vi "Main.vi"() -> ()   [LabVIEW 2017]
uses:
  classes/Scans/Scan.lvclass
  classes/HardwareObjects/DAQ/DAQ.lvclass/DAQ.ctl
  classes/HardwareObjects/Galvonometer/Galvonometer.lvclass/Galvonometer.ctl
  classes/HardwareObjects/Camera/Camera.lvclass/Camera.ctl
  classes/HardwareObjects/PC/PC.lvclass/PC.ctl
  classes/HardwareObjects/Spectrometer/Spectrometer.lvclass/Spectrometer.ctl
  classes/SoftwareObjects/ConfigProc/ConfigProc.lvclass/ConfigProc.ctl
  classes/Scans/Scan.lvclass/Scan.ctl
  classes/HardwareObjects/DAQ/Write Galvo Analog Output Channel(s).vi
  classes/HardwareObjects/Galvonometer/Write Analog Output Channel.vi
  classes/HardwareObjects/Galvonometer/Write Scan Direction.vi
  classes/HardwareObjects/Camera/Write Bit Depth.vi
  classes/HardwareObjects/Camera/Write Camera Dimensions.vi
  classes/HardwareObjects/Camera/Write Data Representation.vi
  classes/HardwareObjects/Camera/Write Duty Cycle.vi
  classes/HardwareObjects/Camera/Write Make, Model.vi
  classes/HardwareObjects/Camera/Write Max Frequency (kHz).vi
  classes/HardwareObjects/Camera/Write Return Time (us).vi
  classes/HardwareObjects/PC/Write Max Number of Cores.vi
  classes/HardwareObjects/PC/Write Path to DLL.vi
  classes/HardwareObjects/DAQ/Write Camera Counter.vi
  classes/HardwareObjects/DAQ/Write Camera Counter Output Terminal.vi
  classes/HardwareObjects/DAQ/Write Galvo Counter.vi
  classes/HardwareObjects/DAQ/Write Galvo Counter Terminal.vi
  classes/HardwareObjects/DAQ/Write Master Counter.vi
  classes/HardwareObjects/DAQ/Write Master Counter Terminal.vi
  classes/HardwareObjects/Spectrometer/Write Bandwidth (nm).vi
  classes/HardwareObjects/Spectrometer/Write Center wavelength (nm).vi
  classes/HardwareObjects/Spectrometer/Write Make Model.vi
  classes/HardwareObjects/Spectrometer/Write Scan depth (mm).vi
  classes/HardwareObjects/Galvonometer/Write Make Model.vi
  classes/HardwareObjects/Galvonometer/Write Max Scan Angle (degrees).vi
  classes/HardwareObjects/Galvonometer/Write Output Scale Factor (V_degrees).vi
  classes/SoftwareObjects/ConfigProc/Write Blur Coefficient.vi
  classes/SoftwareObjects/ConfigProc/Write Blur Int.vi
  classes/SoftwareObjects/ConfigProc/Write Cores.vi
  classes/SoftwareObjects/ConfigProc/Write Interpolation.vi
  classes/SoftwareObjects/ConfigProc/Write Magnification.vi
  classes/SoftwareObjects/ConfigProc/Write Power.vi
  classes/SoftwareObjects/ConfigProc/Write Soften.vi
  classes/Scans/Read X FOV (degrees).vi
  classes/Scans/Read Y FOV (degrees).vi
  classes/HardwareObjects/DAQ/DAQ.lvclass
  classes/HardwareObjects/Galvonometer/Galvonometer.lvclass
  classes/HardwareObjects/Camera/Camera.lvclass
  classes/HardwareObjects/PC/PC.lvclass
  classes/HardwareObjects/Spectrometer/Spectrometer.lvclass
  classes/SoftwareObjects/ConfigProc/ConfigProc.lvclass
panel:
  out "P":dbl[](array[numeric])=[1.0, 2.0, 3.0, 4.0, 5.0, 6.0, 7.0, 8.0, 9.0, 10.0, 11.0, 12.0, 13.0, 14.0, 15.0, 16.0, 17.0, 18.0, 19.0, 20.0, 21.0, 22.0, 23.0, 24.0, 25.0, 26.0, 27.0, 28.0, 29.0, 30.0, 31.0, 32.0, 33.0, 34.0, 35.0, 36.0, 37.0, 38.0, 39.0, 40.0, 41.0, 42.0, 43.0, 44.0, 45.0, 46.0, 47.0, 48.0, 49.0, 50.0, 51.0, 52.0, 53.0, 54.0, 55.0, 56.0, 57.0, 58.0, 59.0, 60.0, 61.0, 62.0, 63.0, 64.0, 65.0, 66.0, 67.0, 68.0, 69.0, 70.0, 71.0, 72.0, 73.0, 74.0, 75.0, 76.0, 77.0, 78.0, 79.0, 80.0, 81.0, 82.0, 83.0, 84.0, 85.0, 86.0, 87.0, 88.0, 89.0, 90.0, 91.0, 92.0, 93.0, 94.0, 95.0, 96.0, 97.0, 98.0, 99.0, 100.0, 101.0, 102.0, 103.0, 104.0, 105.0, 106.0, 107.0, 108.0, 109.0, 110.0, 111.0, 112.0, 113.0, 114.0, 115.0, 116.0, 117.0, 118.0, 119.0, 120.0, 121.0, 122.0, 123.0, 124.0, 125.0, 126.0, 127.0, 128.0, 129.0, 130.0, 131.0, 132.0, 133.0, 134.0, 135.0, 136.0, 137.0, 138.0, 139.0, 140.0, 141.0, 142.0, 143.0, 144.0, 145.0, 146.0, 147.0, 148.0, 149.0, 150.0, 151.0, 152.0, 153.0, 154.0, 155.0, 156.0, 157.0, 158.0, 159.0, 160.0, 161.0, 162.0, 163.0, 164.0, 165.0, 166.0, 167.0, 168.0, 169.0, 170.0, 171.0, 172.0, 173.0, 174.0, 175.0, 176.0, 177.0, 178.0, 179.0, 180.0, 181.0, 182.0, 183.0, 184.0, 185.0, 186.0, 187.0, 188.0, 189.0, 190.0, 191.0, 192.0, 193.0, 194.0, 195.0, 196.0, 197.0, 198.0, 199.0, 200.0, 201.0, 202.0, 203.0, 204.0, 205.0, 206.0, 207.0, 208.0, 209.0, 210.0, 211.0, 212.0, 213.0, 214.0, 215.0, 216.0, 217.0, 218.0, 219.0, 220.0, 221.0, 222.0, 223.0, 224.0, 225.0, 226.0, 227.0, 228.0, 229.0, 230.0, 231.0, 232.0, 233.0, 234.0, 235.0, 236.0, 237.0, 238.0, 239.0, 240.0, 241.0, 242.0, 243.0, 244.0, 245.0, 246.0, 247.0, 248.0, 249.0, 250.0, 251.0, 252.0, 253.0, 254.0, 255.0, 256.0, 257.0, 258.0, 259.0, 260.0, 261.0, 262.0, 263.0, 264.0, 265.0, 266.0, 267.0, 268.0, 269.0, 270.0, 271.0, 272.0, 273.0, 274.0, 275.0, 276.0, 277.0, 278.0, 279.0, 280.0, 281.0, 282.0, 283.0, 284.0, 285.0, 286.0, 287.0, 288.0, 289.0, 290.0, 291.0, 292.0, 293.0, 294.0, 295.0, 296.0, 297.0, 298.0, 299.0, 300.0, 301.0, 302.0, 303.0, 304.0, 305.0, 306.0, 307.0, 308.0, 309.0, 310.0, 311.0, 312.0, 313.0, 314.0, 315.0, 316.0, 317.0, 318.0, 319.0, 320.0, 321.0, 322.0, 323.0, 324.0, 325.0, 326.0, 327.0, 328.0, 329.0, 330.0, 331.0, 332.0, 333.0, 334.0, 335.0, 336.0, 337.0, 338.0, 339.0, 340.0, 341.0, 342.0, 343.0, 344.0, 345.0, 346.0, 347.0, 348.0, 349.0, 350.0, 351.0, 352.0, 353.0, 354.0, 355.0, 356.0, 357.0, 358.0, 359.0, 360.0, 361.0, 362.0, 363.0, 364.0, 365.0, 366.0, 367.0, 368.0, 369.0, 370.0, 371.0, 372.0, 373.0, 374.0, 375.0, 376.0, 377.0, 378.0, 379.0, 380.0, 381.0, 382.0, 383.0, 384.0, 385.0, 386.0, 387.0, 388.0, 389.0, 390.0, 391.0, 392.0, 393.0, 394.0, 395.0, 396.0, 397.0, 398.0, 399.0, 400.0, 401.0, 402.0, 403.0, 404.0, 405.0, 406.0, 407.0, 408.0, 409.0, 410.0, 411.0, 412.0, 413.0, 414.0, 415.0, 416.0, 417.0, 418.0, 419.0, 420.0, 421.0, 422.0, 423.0, 424.0, 425.0, 426.0, 427.0, 428.0, 429.0, 430.0, 431.0, 432.0, 433.0, 434.0, 435.0, 436.0, 437.0, 438.0, 439.0, 440.0, 441.0, 442.0, 443.0, 444.0, 445.0, 446.0, 447.0, 448.0, 449.0, 450.0, 451.0, 452.0, 453.0, 454.0, 455.0, 456.0, 457.0, 458.0, 459.0, 460.0, 461.0, 462.0, 463.0, 464.0, 465.0, 466.0, 467.0, 468.0, 469.0, 470.0, 471.0, 472.0, 473.0, 474.0, 475.0, 476.0, 477.0, 478.0, 479.0, 480.0, 481.0, 482.0, 483.0, 484.0, 485.0, 486.0, 487.0, 488.0, 489.0, 490.0, 491.0, 492.0, 493.0, 494.0, 495.0, 496.0, 497.0, 498.0, 499.0, 500.0, 501.0, 502.0, 503.0, 504.0, 505.0, 506.0, 507.0, 508.0, 509.0, 510.0, 511.0, 512.0, 513.0, 514.0, 515.0, 516.0, 517.0, 518.0, 519.0, 520.0, 521.0, 522.0, 523.0, 524.0, 525.0, 526.0, 527.0, 528.0, 529.0, 530.0, 531.0, 532.0, 533.0, 534.0, 535.0, 536.0, 537.0, 538.0, 539.0, 540.0, 541.0, 542.0, 543.0, 544.0, 545.0, 546.0, 547.0, 548.0, 549.0, 550.0, 551.0, 552.0, 553.0, 554.0, 555.0, 556.0, 557.0, 558.0, 559.0, 560.0, 561.0, 562.0, 563.0, 564.0, 565.0, 566.0, 567.0, 568.0, 569.0, 570.0, 571.0, 572.0, 573.0, 574.0, 575.0, 576.0, 577.0, 578.0, 579.0, 580.0, 581.0, 582.0, 583.0, 584.0, 585.0, 586.0, 587.0, 588.0, 589.0, 590.0, 591.0, 592.0, 593.0, 594.0, 595.0, 596.0, 597.0, 598.0, 599.0, 600.0, 601.0, 602.0, 603.0, 604.0, 605.0, 606.0, 607.0, 608.0, 609.0, 610.0, 611.0, 612.0, 613.0, 614.0, 615.0, 616.0, 617.0, 618.0, 619.0, 620.0, 621.0, 622.0, 623.0, 624.0, 625.0, 626.0, 627.0, 628.0, 629.0, 630.0, 631.0, 632.0, 633.0, 634.0, 635.0, 636.0, 637.0, 638.0, 639.0, 640.0, 641.0, 642.0, 643.0, 644.0, 645.0, 646.0, 647.0, 648.0, 649.0, 650.0, 651.0, 652.0, 653.0, 654.0, 655.0, 656.0, 657.0, 658.0, 659.0, 660.0, 661.0, 662.0, 663.0, 664.0, 665.0, 666.0, 667.0, 668.0, 669.0, 670.0, 671.0, 672.0, 673.0, 674.0, 675.0, 676.0, 677.0, 678.0, 679.0, 680.0, 681.0, 682.0, 683.0, 684.0, 685.0, 686.0, 687.0, 688.0, 689.0, 690.0, 691.0, 692.0, 693.0, 694.0, 695.0, 696.0, 697.0, 698.0, 699.0, 700.0, 701.0, 702.0, 703.0, 704.0, 705.0, 706.0, 707.0, 708.0, 709.0, 710.0, 711.0, 712.0, 713.0, 714.0, 715.0, 716.0, 717.0, 718.0, 719.0, 720.0, 721.0, 722.0, 723.0, 724.0, 725.0, 726.0, 727.0, 728.0, 729.0, 730.0, 731.0, 732.0, 733.0, 734.0, 735.0, 736.0, 737.0, 738.0, 739.0, 740.0, 741.0, 742.0, 743.0, 744.0, 745.0, 746.0, 747.0, 748.0, 749.0, 750.0, 751.0, 752.0, 753.0, 754.0, 755.0, 756.0, 757.0, 758.0, 759.0, 760.0, 761.0, 762.0, 763.0, 764.0, 765.0, 766.0, 767.0, 768.0, 769.0, 770.0, 771.0, 772.0, 773.0, 774.0, 775.0, 776.0, 777.0, 778.0, 779.0, 780.0, 781.0, 782.0, 783.0, 784.0, 785.0, 786.0, 787.0, 788.0, 789.0, 790.0, 791.0, 792.0, 793.0, 794.0, 795.0, 796.0, 797.0, 798.0, 799.0, 800.0, 801.0, 802.0, 803.0, 804.0, 805.0, 806.0, 807.0, 808.0, 809.0, 810.0, 811.0, 812.0, 813.0, 814.0, 815.0, 816.0, 817.0, 818.0, 819.0, 820.0, 821.0, 822.0, 823.0, 824.0, 825.0, 826.0, 827.0, 828.0, 829.0, 830.0, 831.0, 832.0, 833.0, 834.0, 835.0, 836.0, 837.0, 838.0, 839.0, 840.0, 841.0, 842.0, 843.0, 844.0, 845.0, 846.0, 847.0, 848.0, 849.0, 850.0, 851.0, 852.0, 853.0, 854.0, 855.0, 856.0, 857.0, 858.0, 859.0, 860.0, 861.0, 862.0, 863.0, 864.0, 865.0, 866.0, 867.0, 868.0, 869.0, 870.0, 871.0, 872.0, 873.0, 874.0, 875.0, 876.0, 877.0, 878.0, 879.0, 880.0, 881.0, 882.0, 883.0, 884.0, 885.0, 886.0, 887.0, 888.0, 889.0, 890.0, 891.0, 892.0, 893.0, 894.0, 895.0, 896.0, 897.0, 898.0, 899.0, 900.0, 901.0, 902.0, 903.0, 904.0, 905.0, 906.0, 907.0, 908.0, 909.0, 910.0, 911.0, 912.0, 913.0, 914.0, 915.0, 916.0, 917.0, 918.0, 919.0, 920.0, 921.0, 922.0, 923.0, 924.0, 925.0, 926.0, 927.0, 928.0, 929.0, 930.0, 931.0, 932.0, 933.0, 934.0, 935.0, 936.0, 937.0, 938.0, 939.0, 940.0, 941.0, 942.0, 943.0, 944.0, 945.0, 946.0, 947.0, 948.0, 949.0, 950.0, 951.0, 952.0, 953.0, 954.0, 955.0, 956.0, 957.0, 958.0, 959.0, 960.0, 961.0, 962.0, 963.0, 964.0, 965.0, 966.0, 967.0, 968.0, 969.0, 970.0, 971.0, 972.0, 973.0, 974.0, 975.0, 976.0, 977.0, 978.0, 979.0, 980.0, 981.0, 982.0, 983.0, 984.0, 985.0, 986.0, 987.0, 988.0, 989.0, 990.0, 991.0, 992.0, 993.0, 994.0, 995.0, 996.0, 997.0, 998.0, 999.0, 1000.0, 1001.0, 1002.0, 1003.0, 1004.0, 1005.0, 1006.0, 1007.0, 1008.0, 1009.0, 1010.0, 1011.0, 1012.0, 1013.0, 1014.0, 1015.0, 1016.0, 1017.0, 1018.0, 1019.0, 1020.0, 1021.0, 1022.0, 1023.0, 1024.0, 1025.0, 1026.0, 1027.0, 1028.0, 1029.0, 1030.0, 1031.0, 1032.0, 1033.0, 1034.0, 1035.0, 1036.0, 1037.0, 1038.0, 1039.0, 1040.0, 1041.0, 1042.0, 1043.0, 1044.0, 1045.0, 1046.0, 1047.0, 1048.0, 1049.0, 1050.0, 1051.0, 1052.0, 1053.0, 1054.0, 1055.0, 1056.0, 1057.0, 1058.0, 1059.0, 1060.0, 1061.0, 1062.0, 1063.0, 1064.0, 1065.0, 1066.0, 1067.0, 1068.0, 1069.0, 1070.0, 1071.0, 1072.0, 1073.0, 1074.0, 1075.0, 1076.0, 1077.0, 1078.0, 1079.0, 1080.0, 1081.0, 1082.0, 1083.0, 1084.0, 1085.0, 1086.0, 1087.0, 1088.0, 1089.0, 1090.0, 1091.0, 1092.0, 1093.0, 1094.0, 1095.0, 1096.0, 1097.0, 1098.0, 1099.0, 1100.0, 1101.0, 1102.0, 1103.0, 1104.0, 1105.0, 1106.0, 1107.0, 1108.0, 1109.0, 1110.0, 1111.0, 1112.0, 1113.0, 1114.0, 1115.0, 1116.0, 1117.0, 1118.0, 1119.0, 1120.0, 1121.0, 1122.0, 1123.0, 1124.0, 1125.0, 1126.0, 1127.0, 1128.0, 1129.0, 1130.0, 1131.0, 1132.0, 1133.0, 1134.0, 1135.0, 1136.0, 1137.0, 1138.0, 1139.0, 1140.0, 1141.0, 1142.0, 1143.0, 1144.0, 1145.0, 1146.0, 1147.0, 1148.0, 1149.0, 1150.0, 1151.0, 1152.0, 1153.0, 1154.0, 1155.0, 1156.0, 1157.0, 1158.0, 1159.0, 1160.0, 1161.0, 1162.0, 1163.0, 1164.0, 1165.0, 1166.0, 1167.0, 1168.0, 1169.0, 1170.0, 1171.0, 1172.0, 1173.0, 1174.0, 1175.0, 1176.0, 1177.0, 1178.0, 1179.0, 1180.0, 1181.0, 1182.0, 1183.0, 1184.0, 1185.0, 1186.0, 1187.0, 1188.0, 1189.0, 1190.0, 1191.0, 1192.0, 1193.0, 1194.0, 1195.0, 1196.0, 1197.0, 1198.0, 1199.0, 1200.0, 1201.0, 1202.0, 1203.0, 1204.0, 1205.0, 1206.0, 1207.0, 1208.0, 1209.0, 1210.0, 1211.0, 1212.0, 1213.0, 1214.0, 1215.0, 1216.0, 1217.0, 1218.0, 1219.0, 1220.0, 1221.0, 1222.0, 1223.0, 1224.0, 1225.0, 1226.0, 1227.0, 1228.0, 1229.0, 1230.0, 1231.0, 1232.0, 1233.0, 1234.0, 1235.0, 1236.0, 1237.0, 1238.0, 1239.0, 1240.0, 1241.0, 1242.0, 1243.0, 1244.0, 1245.0, 1246.0, 1247.0, 1248.0, 1249.0, 1250.0, 1251.0, 1252.0, 1253.0, 1254.0, 1255.0, 1256.0, 1257.0, 1258.0, 1259.0, 1260.0, 1261.0, 1262.0, 1263.0, 1264.0, 1265.0, 1266.0, 1267.0, 1268.0, 1269.0, 1270.0, 1271.0, 1272.0, 1273.0, 1274.0, 1275.0, 1276.0, 1277.0, 1278.0, 1279.0, 1280.0, 1281.0, 1282.0, 1283.0, 1284.0, 1285.0, 1286.0, 1287.0, 1288.0, 1289.0, 1290.0, 1291.0, 1292.0, 1293.0, 1294.0, 1295.0, 1296.0, 1297.0, 1298.0, 1299.0, 1300.0, 1301.0, 1302.0, 1303.0, 1304.0, 1305.0, 1306.0, 1307.0, 1308.0, 1309.0, 1310.0, 1311.0, 1312.0, 1313.0, 1314.0, 1315.0, 1316.0, 1317.0, 1318.0, 1319.0, 1320.0, 1321.0, 1322.0, 1323.0, 1324.0, 1325.0, 1326.0, 1327.0, 1328.0, 1329.0, 1330.0, 1331.0, 1332.0, 1333.0, 1334.0, 1335.0, 1336.0, 1337.0, 1338.0, 1339.0, 1340.0, 1341.0, 1342.0, 1343.0, 1344.0, 1345.0, 1346.0, 1347.0, 1348.0, 1349.0, 1350.0, 1351.0, 1352.0, 1353.0, 1354.0, 1355.0, 1356.0, 1357.0, 1358.0, 1359.0, 1360.0, 1361.0, 1362.0, 1363.0, 1364.0, 1365.0, 1366.0, 1367.0, 1368.0, 1369.0, 1370.0, 1371.0, 1372.0, 1373.0, 1374.0, 1375.0, 1376.0, 1377.0, 1378.0, 1379.0, 1380.0, 1381.0, 1382.0, 1383.0, 1384.0, 1385.0, 1386.0, 1387.0, 1388.0, 1389.0, 1390.0, 1391.0, 1392.0, 1393.0, 1394.0, 1395.0, 1396.0, 1397.0, 1398.0, 1399.0, 1400.0, 1401.0, 1402.0, 1403.0, 1404.0, 1405.0, 1406.0, 1407.0, 1408.0, 1409.0, 1410.0, 1411.0, 1412.0, 1413.0, 1414.0, 1415.0, 1416.0, 1417.0, 1418.0, 1419.0, 1420.0, 1421.0, 1422.0, 1423.0, 1424.0, 1425.0, 1426.0, 1427.0, 1428.0, 1429.0, 1430.0, 1431.0, 1432.0, 1433.0, 1434.0, 1435.0, 1436.0, 1437.0, 1438.0, 1439.0, 1440.0, 1441.0, 1442.0, 1443.0, 1444.0, 1445.0, 1446.0, 1447.0, 1448.0, 1449.0, 1450.0, 1451.0, 1452.0, 1453.0, 1454.0, 1455.0, 1456.0, 1457.0, 1458.0, 1459.0, 1460.0, 1461.0, 1462.0, 1463.0, 1464.0, 1465.0, 1466.0, 1467.0, 1468.0, 1469.0, 1470.0, 1471.0, 1472.0, 1473.0, 1474.0, 1475.0, 1476.0, 1477.0, 1478.0, 1479.0, 1480.0, 1481.0, 1482.0, 1483.0, 1484.0, 1485.0, 1486.0, 1487.0, 1488.0, 1489.0, 1490.0, 1491.0, 1492.0, 1493.0, 1494.0, 1495.0, 1496.0, 1497.0, 1498.0, 1499.0, 1500.0, 1501.0, 1502.0, 1503.0, 1504.0, 1505.0, 1506.0, 1507.0, 1508.0, 1509.0, 1510.0, 1511.0, 1512.0, 1513.0, 1514.0, 1515.0, 1516.0, 1517.0, 1518.0, 1519.0, 1520.0, 1521.0, 1522.0, 1523.0, 1524.0, 1525.0, 1526.0, 1527.0, 1528.0, 1529.0, 1530.0, 1531.0, 1532.0, 1533.0, 1534.0, 1535.0, 1536.0, 1537.0, 1538.0, 1539.0, 1540.0, 1541.0, 1542.0, 1543.0, 1544.0, 1545.0, 1546.0, 1547.0, 1548.0, 1549.0, 1550.0, 1551.0, 1552.0, 1553.0, 1554.0, 1555.0, 1556.0, 1557.0, 1558.0, 1559.0, 1560.0, 1561.0, 1562.0, 1563.0, 1564.0, 1565.0, 1566.0, 1567.0, 1568.0, 1569.0, 1570.0, 1571.0, 1572.0, 1573.0, 1574.0, 1575.0, 1576.0, 1577.0, 1578.0, 1579.0, 1580.0, 1581.0, 1582.0, 1583.0, 1584.0, 1585.0, 1586.0, 1587.0, 1588.0, 1589.0, 1590.0, 1591.0, 1592.0, 1593.0, 1594.0, 1595.0, 1596.0, 1597.0, 1598.0, 1599.0, 1600.0, 1601.0, 1602.0, 1603.0, 1604.0, 1605.0, 1606.0, 1607.0, 1608.0, 1609.0, 1610.0, 1611.0, 1612.0, 1613.0, 1614.0, 1615.0, 1616.0, 1617.0, 1618.0, 1619.0, 1620.0, 1621.0, 1622.0, 1623.0, 1624.0, 1625.0, 1626.0, 1627.0, 1628.0, 1629.0, 1630.0, 1631.0, 1632.0, 1633.0, 1634.0, 1635.0, 1636.0, 1637.0, 1638.0, 1639.0, 1640.0, 1641.0, 1642.0, 1643.0, 1644.0, 1645.0, 1646.0, 1647.0, 1648.0, 1649.0, 1650.0, 1651.0, 1652.0, 1653.0, 1654.0, 1655.0, 1656.0, 1657.0, 1658.0, 1659.0, 1660.0, 1661.0, 1662.0, 1663.0, 1664.0, 1665.0, 1666.0, 1667.0, 1668.0, 1669.0, 1670.0, 1671.0, 1672.0, 1673.0, 1674.0, 1675.0, 1676.0, 1677.0, 1678.0, 1679.0, 1680.0, 1681.0, 1682.0, 1683.0, 1684.0, 1685.0, 1686.0, 1687.0, 1688.0, 1689.0, 1690.0, 1691.0, 1692.0, 1693.0, 1694.0, 1695.0, 1696.0, 1697.0, 1698.0, 1699.0, 1700.0, 1701.0, 1702.0, 1703.0, 1704.0, 1705.0, 1706.0, 1707.0, 1708.0, 1709.0, 1710.0, 1711.0, 1712.0, 1713.0, 1714.0, 1715.0, 1716.0, 1717.0, 1718.0, 1719.0, 1720.0, 1721.0, 1722.0, 1723.0, 1724.0, 1725.0, 1726.0, 1727.0, 1728.0, 1729.0, 1730.0, 1731.0, 1732.0, 1733.0, 1734.0, 1735.0, 1736.0, 1737.0, 1738.0, 1739.0, 1740.0, 1741.0, 1742.0, 1743.0, 1744.0, 1745.0, 1746.0, 1747.0, 1748.0, 1749.0, 1750.0, 1751.0, 1752.0, 1753.0, 1754.0, 1755.0, 1756.0, 1757.0, 1758.0, 1759.0, 1760.0, 1761.0, 1762.0, 1763.0, 1764.0, 1765.0, 1766.0, 1767.0, 1768.0, 1769.0, 1770.0, 1771.0, 1772.0, 1773.0, 1774.0, 1775.0, 1776.0, 1777.0, 1778.0, 1779.0, 1780.0, 1781.0, 1782.0, 1783.0, 1784.0, 1785.0, 1786.0, 1787.0, 1788.0, 1789.0, 1790.0, 1791.0, 1792.0, 1793.0, 1794.0, 1795.0, 1796.0, 1797.0, 1798.0, 1799.0, 1800.0, 1801.0, 1802.0, 1803.0, 1804.0, 1805.0, 1806.0, 1807.0, 1808.0, 1809.0, 1810.0, 1811.0, 1812.0, 1813.0, 1814.0, 1815.0, 1816.0, 1817.0, 1818.0, 1819.0, 1820.0, 1821.0, 1822.0, 1823.0, 1824.0, 1825.0, 1826.0, 1827.0, 1828.0, 1829.0, 1830.0, 1831.0, 1832.0, 1833.0, 1834.0, 1835.0, 1836.0, 1837.0, 1838.0, 1839.0, 1840.0, 1841.0, 1842.0, 1843.0, 1844.0, 1845.0, 1846.0, 1847.0, 1848.0, 1849.0, 1850.0, 1851.0, 1852.0, 1853.0, 1854.0, 1855.0, 1856.0, 1857.0, 1858.0, 1859.0, 1860.0, 1861.0, 1862.0, 1863.0, 1864.0, 1865.0, 1866.0, 1867.0, 1868.0, 1869.0, 1870.0, 1871.0, 1872.0, 1873.0, 1874.0, 1875.0, 1876.0, 1877.0, 1878.0, 1879.0, 1880.0, 1881.0, 1882.0, 1883.0, 1884.0, 1885.0, 1886.0, 1887.0, 1888.0, 1889.0, 1890.0, 1891.0, 1892.0, 1893.0, 1894.0, 1895.0, 1896.0, 1897.0, 1898.0, 1899.0, 1900.0, 1901.0, 1902.0, 1903.0, 1904.0, 1905.0, 1906.0, 1907.0, 1908.0, 1909.0, 1910.0, 1911.0, 1912.0, 1913.0, 1914.0, 1915.0, 1916.0, 1917.0, 1918.0, 1919.0, 1920.0, 1921.0, 1922.0, 1923.0, 1924.0, 1925.0, 1926.0, 1927.0, 1928.0, 1929.0, 1930.0, 1931.0, 1932.0, 1933.0, 1934.0, 1935.0, 1936.0, 1937.0, 1938.0, 1939.0, 1940.0, 1941.0, 1942.0, 1943.0, 1944.0, 1945.0, 1946.0, 1947.0, 1948.0, 1949.0, 1950.0, 1951.0, 1952.0, 1953.0, 1954.0, 1955.0, 1956.0, 1957.0, 1958.0, 1959.0, 1960.0, 1961.0, 1962.0, 1963.0, 1964.0, 1965.0, 1966.0, 1967.0, 1968.0, 1969.0, 1970.0, 1971.0, 1972.0, 1973.0, 1974.0, 1975.0, 1976.0, 1977.0, 1978.0, 1979.0, 1980.0, 1981.0, 1982.0, 1983.0, 1984.0, 1985.0, 1986.0, 1987.0, 1988.0, 1989.0, 1990.0, 1991.0, 1992.0, 1993.0, 1994.0, 1995.0, 1996.0, 1997.0, 1998.0, 1999.0, 2000.0, 2001.0, 2002.0, 2003.0, 2004.0, 2005.0, 2006.0, 2007.0, 2008.0, 2009.0, 2010.0, 2011.0, 2012.0, 2013.0, 2014.0, 2015.0, 2016.0, 2017.0, 2018.0, 2019.0, 2020.0, 2021.0, 2022.0, 2023.0, 2024.0, 2025.0, 2026.0, 2027.0, 2028.0, 2029.0, 2030.0, 2031.0, 2032.0, 2033.0, 2034.0, 2035.0, 2036.0, 2037.0, 2038.0, 2039.0, 2040.0, 2041.0, 2042.0, 2043.0, 2044.0, 2045.0, 2046.0, 2047.0, 2048.0]
  out "Gc":cdb[](array[numeric])
  out "Mean intensity per pixel":cluster{"Ramp Pattern":dbl[], dbl[]}[](graph)=[{"Ramp Pattern"=array[2048 elements], array[2048 elements]}, {"Ramp Pattern"=[767.5, 767.5], [0.0, 100.0]}, {"Ramp Pattern"=[932.5, 932.5], [0.0, 100.0]}, {"Ramp Pattern"=[850.0, 850.0], [0.0, 100.0]}]
  out "cropLinesOut":dbl
  in  "Skip Processing":bool
  out "wavenumber vector":dbl[](array[numeric])
  out "Max file size exceeded":bool
  out "Progress":cluster{"wb":sgl, "wb txt":string} {"wb" scale=0.0..1.0}
  in  "Save Settings":bool
  in  "Skip FFT":bool
  in  "Adv. Settings":T1(tab)
  out "Other error":errorcluster
  out "Initialization Error":errorcluster
  in  "Hardware Tabs":T2(tab)
  in  "Camera Ctrl":T3={"Bit Depth"=10.0, "Duty Cycle"=0.95, "Data Representation"=enum."U16", "Max Frequency (kHz)"=130.0, "Return Time (µs)"=0.0, "Make, Model"="Wasatch Cobra S800", "Camera Dimensions (px)"=[]}
  in  "PC Ctrl":T4={"Max Number of Cores"=8.0, "Path to DLL"=path ""}
  in  "DAQ Ctrl":T5={"Camera Counter"="Dev1/ctr1", "Camera Counter PFI"="/Dev1/PFI2", "Galvo Counter"="Dev1/ctr2", "Galvo Counter PFI"="/Dev1/PFI1", "Master Counter"="Dev1/ctr0", "Master Counter PFI"="/Dev1/PFI0", "Galvo Analog Output Channel(s)"="Dev1/ao0:1"}
  in  "Spec Ctrl":T6={"Bandwidth (nm)"=0.0, "Center wavelength (nm)"=0.0, "Make Model"="", "Scan depth (mm)"=2.0}
  in  "Galvo Ctrl":T7
  in  "Processing Tabs":T8(tab)
  in  "Display Ctrl":cluster{"I'=Log_10(I)":bool}
  in  "Fourier Ctrl":T9={"Blur Coefficient"=0.0, "Blur Int"=0.0, "Cores to Use"=8.0, "Interpolation"=1.0, "Magnification"=1.0, "Power"=1.0, "Soften"=0.0, "Weight"=[]}
  in  "Optimize DispComp":bool
  in  "Dispersion Ctrl":cluster{"C2":dbl, "C3":dbl}
  in  "File Ctrl":T10={"Subject ID"="noise", "Eye"=FALSE, "Output Path"=path "E:/", "String"="OS", "String 2"="OD"}
  out "Current Scan Schematic":cluster{dbl[], dbl[]}[](graph)=[{[-10.0, 10.0, 10.0, -10.0, -10.0], [10.0, 10.0, -10.0, -10.0, 10.0]}, {[-12.5, 12.5, 12.5, -12.5, -12.5], [12.5, 12.5, -12.5, -12.5, 12.5]}]
  out "Stopping":bool
  in  "Stop":bool
  in  "Reset":bool
  in  "Save":bool
  out "Saving":bool
  out "Depth":dbl[][](graph)
  out "Time (s)":sgl=130.0 format="%#_3g"
  out "Memory (GB)":dbl format="%#_3g"
  out "Exceeds Max Voltage":bool
  in  "Scan Settings":T11={"A Scans"=500, "B Scans"=500, "Repeat B Scans"=1, "C Scans"=1.0, "X FOV (°)"=10.0, "Y FOV (°)"=10.0, "Rotate Scan (°)"=0.0, "X Offset (°)"=0.0, "Y Offset (°)"=0.0, "Bidirectional\nScanning"=FALSE, "Raster Type"="Rectangle", "Angio Mode"="None"} {"Y FOV (°)" min=0.0 max=20.0 step=0.5; "Repeat B Scans" min=1 step=1; "C Scans" min=1.0 step=1.0; "B Scans" min=1 step=1; "A Scans" min=1 max=1023 step=10; "Rotate Scan (°)" min=0.0 max=360.0 step=90.0; "X FOV (°)" min=0.0 max=20.0 step=0.5}
  # "Press Apply to apply setting changes"
  # "exp(i*C2*(k-k0)^2 + C3*(k-k0)^3)"
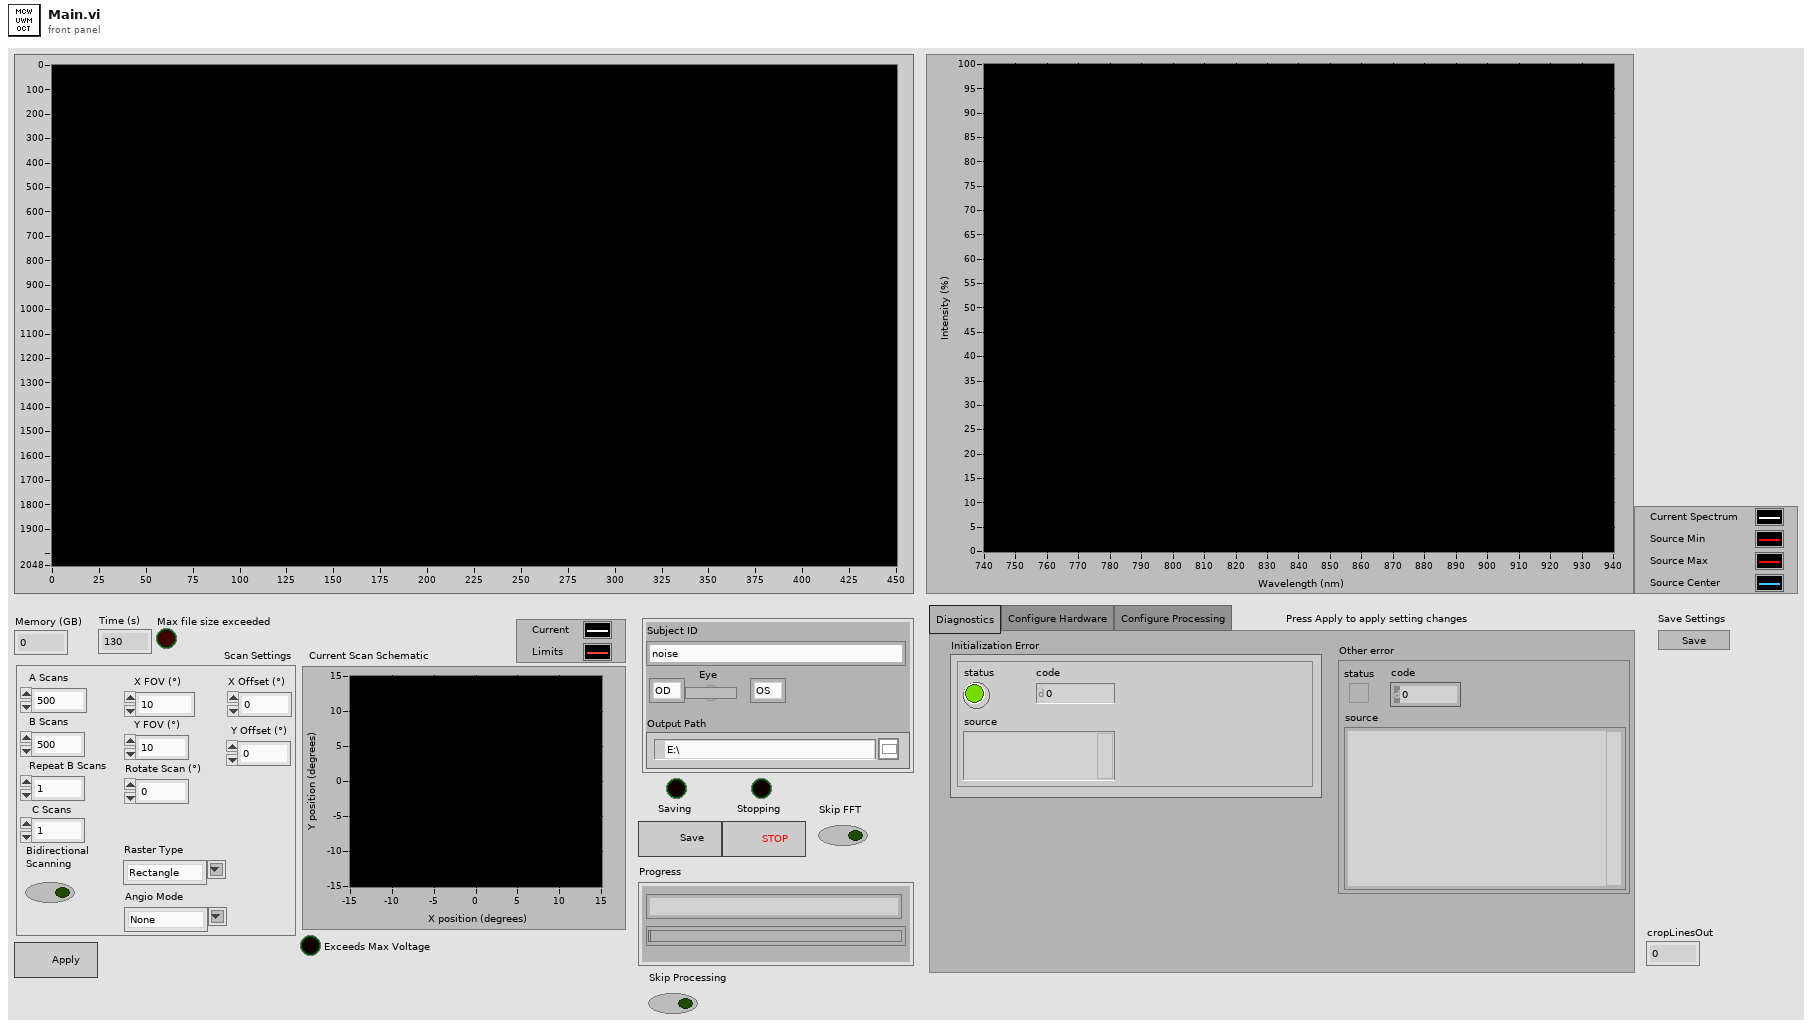
[diagram p1: front panel]
types:
  T1 = enum32{"Diagnostics", "Configure Hardware", "Configure Processing"}
  T2 = enum32{"Camera", "PC", "DAQ", "Laser", "Spectrometer", "Galvos"}
  T3 = cluster{"Bit Depth":dbl, "Duty Cycle":sgl, "Data Representation":enum16{"U8", "I8", "U16", "I16"}, "Max Frequency (kHz)":sgl, "Return Time (µs)":sgl, "Make, Model":string, "Camera Dimensions (px)":u16[]}
  T4 = cluster{"Max Number of Cores":dbl, "Path to DLL":path}
  T5 = cluster{"Camera Counter":tag, "Camera Counter PFI":tag, "Galvo Counter":tag, "Galvo Counter PFI":tag, "Master Counter":tag, "Master Counter PFI":tag, "Galvo Analog Output Channel(s)":tag}
  T6 = cluster{"Bandwidth (nm)":dbl, "Center wavelength (nm)":dbl, "Make Model":string, "Scan depth (mm)":dbl}
  T7 = cluster{"Max Scan Angle (degrees)":dbl, "Output Scale Factor (V/degree)":dbl, "Make Model":string}
  T8 = enum32{"Display Intensity Mapping", "Fourier Transform", "Dispersion"}
  T9 = cluster{"Blur Coefficient":dbl, "Blur Int":dbl, "Cores to Use":dbl, "Interpolation":dbl, "Magnification":dbl, "Power":dbl, "Soften":dbl, "Weight":cdb[][]}
  T10 = cluster{"Subject ID":string, "Eye":bool, "Output Path":path, "String":string, "String 2":string}
  T11 = cluster{"A Scans":u32, "B Scans":u32, "Repeat B Scans":u32, "C Scans":dbl, "X FOV (°)":dbl, "Y FOV (°)":dbl, "Rotate Scan (°)":dbl, "X Offset (°)":dbl, "Y Offset (°)":dbl, "Bidirectional\nScanning":bool, "Raster Type":string, "Angio Mode":string}
  T12 = cluster{"Spectrometer out":refnum<class "Spectrometer.lvclass">, "Camera out":refnum<class "Camera.lvclass">, "DAQ out":refnum<class "DAQ.lvclass">, refnum<class "Galvonometer.lvclass">[], "PC out":refnum<class "PC.lvclass">, "Proc out":refnum<class "ConfigProc.lvclass">}
  T13 = cluster{"Camera Ctrl":cluster{"Bit Depth":dbl, "Duty Cycle":sgl, "Data Representation":enum16{"U8", "I8", "U16", "I16"}, "Max Frequency (kHz)":sgl, "Return Time (µs)":sgl, "Make, Model":string, "Camera Dimensions (px)":u16[]}, "PC Ctrl":cluster{"Max Number of Cores":dbl, "Path to DLL":path}, "DAQ Ctrl":cluster{"Camera Counter":tag, "Camera Counter PFI":tag, "Galvo Counter":tag, "Galvo Counter PFI":tag, "Master Counter":tag, "Master Counter PFI":tag, "Galvo Analog Output Channel(s)":tag}, "Spec Ctrl":cluster{"Bandwidth (nm)":dbl, "Center wavelength (nm)":dbl, "Make Model":string, "Scan depth (mm)":dbl}, "Galvo Ctrl":cluster{"Max Scan Angle (degrees)":dbl, "Output Scale Factor (V/degree)":dbl, "Make Model":string}}
  T14 = cluster{"Fourier Ctrl":cluster{"Blur Coefficient":dbl, "Blur Int":dbl, "Cores to Use":dbl, "Interpolation":dbl, "Magnification":dbl, "Power":dbl, "Soften":dbl, "Weight":cdb[][]}, "Display Ctrl":cluster{"I'=Log_10(I)":bool}, "Dispersion Ctrl":cluster{"C2":dbl, "C3":dbl}}
  T15 = enum8{"Enabled", "Disabled", "Disabled and Grayed Out"}
  T16 = cluster{"Def Spectrometer":refnum<class "Spectrometer.lvclass">, "Def Camera":refnum<class "Camera.lvclass">, "Def DAQ":refnum<class "DAQ.lvclass">, "Array":refnum<class "Galvonometer.lvclass">[], "Def PC":refnum<class "PC.lvclass">, "Def Proc":refnum<class "ConfigProc.lvclass">}
  T17 = cluster{"A scans":dbl, "Pixel Count":u16, dbl[][], cdb[][]}
  T18 = typedef "IMAQ Image.ctl" = refnum<image>
  T19 = cluster{"IMAQ Session Out":refnum<k11>, T18[], "New Image":T18}
  T20 = cluster{"IMAQ Session Out":refnum<k11>, "Array":T18[], "New Image":T18}
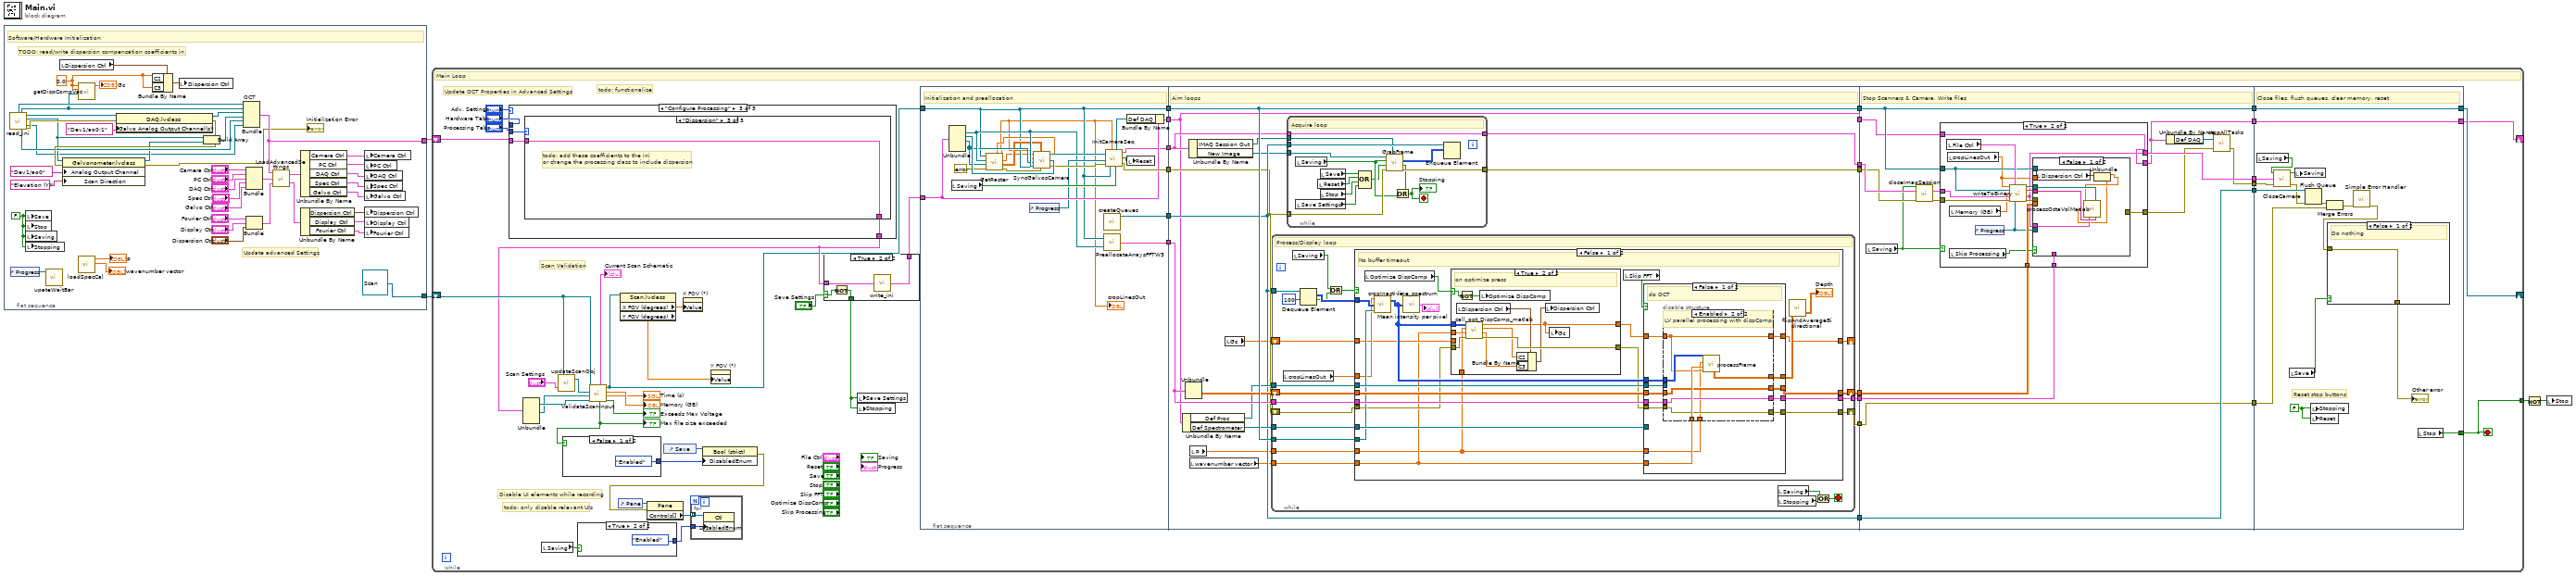
[diagram p0: block diagram]
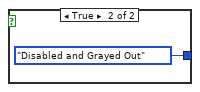
[diagram p2: hidden frame]
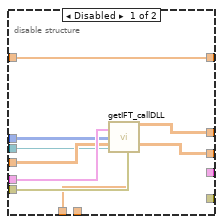
[diagram p4: hidden frame]
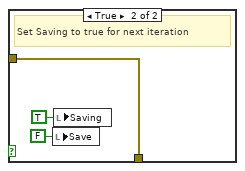
[diagram p9: hidden frame]
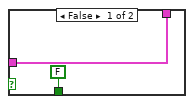
[diagram p10: hidden frame]
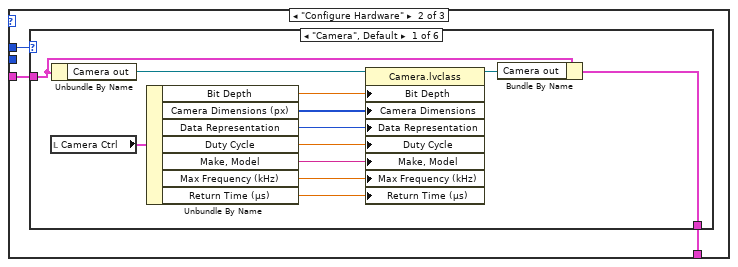
[diagram p12: hidden frame]
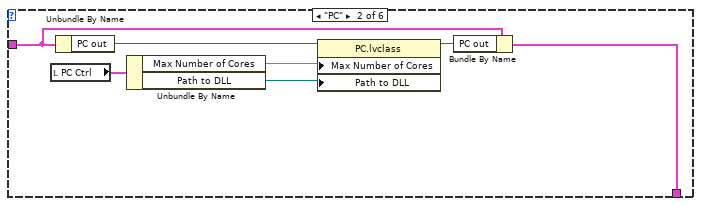
[diagram p13: hidden frame]
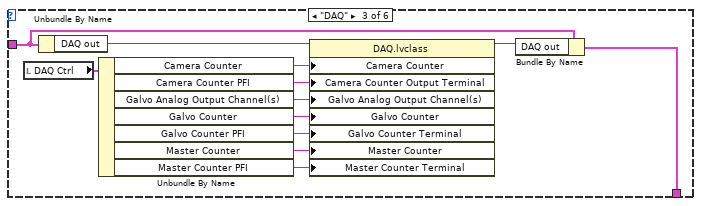
[diagram p14: hidden frame]
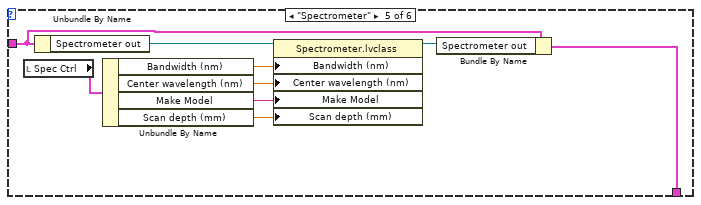
[diagram p16: hidden frame]
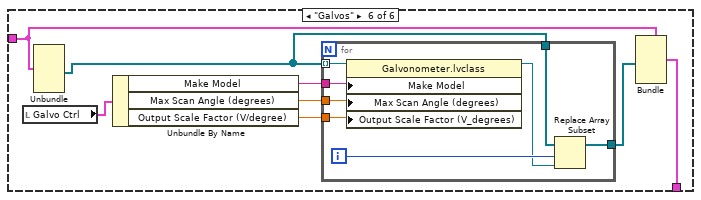
[diagram p17: hidden frame]
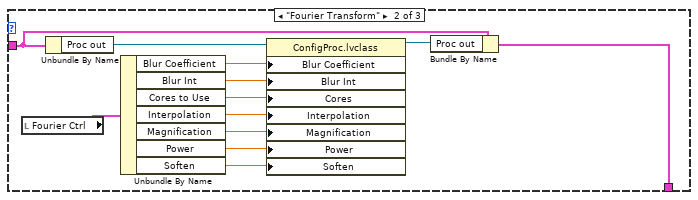
[diagram p19: hidden frame]
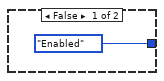
[diagram p20: hidden frame]
diagram:
  n1 = flat-sequence {
    tunnel: [w33] -> w4
    tunnel: [refnum<class "Scan.lvclass"> refnum ("Def Scan")] -> w3
    frame #0 {
      w8 = 0.0 ("C2")
      w16 = FALSE
      # "TODO: read/write dispersion compensation coefficients in"
      # "Update advanced Settings"
      # "Software/Hardware Initialization"
      n2 = call "read_ini.vi"() -> ("Spectrometer out"=w24:refnum<class "Spectrometer.lvclass">, "Camera out"=w11:refnum<class "Camera.lvclass">, "DAQ out"=w23:refnum<class "DAQ.lvclass">, "Galvo out"=w21:refnum<class "Galvonometer.lvclass">, "Proc out"=w13:refnum<class "ConfigProc.lvclass">, "PC out"=w22:refnum<class "PC.lvclass">, "error out"=w48:errorcluster)  [unwired: 9 in]
      n3 = control-ref of="Progress"() -> (w12:refnum<vi>)
      n4 = local write "Save"(w16) -> ()
      n5 = local write "Stop"(w16) -> ()
      n6 = local write "Saving"(w16) -> ()
      n7 = local write "Stopping"(w16) -> ()
      n8 = call "upateWaitBar.vi"("Progress"=w12) -> ()  [unwired: 4 in, 1 out]
      n9 = local read "Dispersion Ctrl"() -> (w10:cluster{"C2":dbl, "C3":dbl})
      n10 = call "loadSpecCal.vi"() -> ("interp_index"=→"wavenumber vector":dbl[], "P"=→"P":dbl[])  [unwired: 10 in]
      n11 = call "getDispCompVec.vi"("Camera in"=w11, "C3"=w8, "C2"=w8) -> ("Gc"=→"Gc":cdb[])  [unwired: 8 in]
      n12 = property class="DAQ.lvclass"(reference=w23, error in=w48, "Galvo Analog Output Channel(s)"=tag "Dev1/ao0:1") -> (reference out=w46:refnum<class "DAQ.lvclass">, error out=w49:errorcluster)
      n13 = property class="Galvonometer.lvclass"(reference=w21, error in=w49, "Analog Output Channel"=tag "Dev1/ao0", "Scan Direction"="Elevation (Y)") -> (reference out=w18:refnum<class "Galvonometer.lvclass">, error out=→"Initialization Error":errorcluster)
      n14 = Bundle By Name(cluster=w10, "C2"=w8, "C3"=w8) -> (w9:cluster{"C2":dbl, "C3":dbl})
      n15 = local write "Dispersion Ctrl"(w9) -> ()
      n16 = Build Array(w21, w18) -> (w47:refnum<class "Galvonometer.lvclass">[])
      n17 = Bundle "OCT"("Spectrometer out"=w24, "Camera out"=w11, "DAQ out"=w46, w47, "PC out"=w22, "Proc out"=w13) -> (w33:T12)  [unwired: 1 in]
      n18 = Bundle("Camera Ctrl"="Camera Ctrl", "PC Ctrl"="PC Ctrl", "DAQ Ctrl"="DAQ Ctrl", "Spec Ctrl"="Spec Ctrl", "Galvo Ctrl"="Galvo Ctrl") -> (w35:T13)  [unwired: 1 in]
      n19 = Bundle("Fourier Ctrl"="Fourier Ctrl", "Display Ctrl"="Display Ctrl", "Dispersion Ctrl"="Dispersion Ctrl") -> (w14:T14)  [unwired: 1 in]
      n20 = call "LoadAdvancedSettings.vi"("Software settings in"=w14, "Hardware settings in"=w35, "OCT in"=w33) -> ("Software settings out"=w27:T14, "Hardware  settings out"=w34:T13)
      n21 = Unbundle By Name(w34) -> ("Camera Ctrl"=w32:T3, "PC Ctrl"=w31:T4, "DAQ Ctrl"=w30:T5, "Spec Ctrl"=w29:T6, "Galvo Ctrl"=w28:T7)
      n22 = Unbundle By Name(w27) -> ("Dispersion Ctrl"=w26:cluster{"C2":dbl, "C3":dbl}, "Display Ctrl"=w25:cluster{"I'=Log_10(I)":bool}, "Fourier Ctrl"=w15:T9)
      n23 = local write "Camera Ctrl"(w32) -> ()
      n24 = local write "PC Ctrl"(w31) -> ()
      n25 = local write "DAQ Ctrl"(w30) -> ()
      n26 = local write "Spec Ctrl"(w29) -> ()
      n27 = local write "Galvo Ctrl"(w28) -> ()
      n28 = local write "Dispersion Ctrl"(w26) -> ()
      n29 = local write "Display Ctrl"(w25) -> ()
      n30 = local write "Fourier Ctrl"(w15) -> ()
    }
  }
  n31 = while {
    shift-right: [w88] -> _
    shift-left: w3 -> [w87]
    tunnel: [w52] -> w1
    shift-right: [w50] -> _
    shift-left: w4 -> [w80]
    stop <- w52 stop-if-true
    # "todo: only disable relevant UIs"
    # "todo: functionalize"
    # "Disable UI elements while recording"
    # "Scan Validation"
    # "Update OCT Properties in Advanced Settings"
    # "Main Loop"
    n32 = case shown="\"Configure Processing\"" "Adv. Settings" {
      tunnel: "Hardware Tabs" -> [_ w331 _]
      tunnel: w80 -> [w328 w330 w390]
      tunnel: "Processing Tabs" -> [_ _ w391]
      tunnel: [w328 w329 w389] -> w77
      frame "Diagnostics", Default {
      }
      frame "Configure Hardware" {
        n33 = case shown="\"Camera\", Default" w331 {
          tunnel: w330 -> [w334 w350 w362 w363 w372 w380]
          tunnel: [w333 w344 w361 w363 w365 w373] -> w329
          frame "Camera", Default {
            n34 = local read "Camera Ctrl"() -> (w342:T3)
            n35 = Unbundle By Name(w334) -> ("Camera out"=w343:refnum<class "Camera.lvclass">)
            n36 = Unbundle By Name(w342) -> ("Bit Depth"=w341:dbl, "Camera Dimensions (px)"=w340:u16[], "Data Representation"=w339:enum16{"U8", "I8", "U16", "I16"}, "Duty Cycle"=w338:sgl, "Make, Model"=w337:string, "Max Frequency (kHz)"=w336:sgl, "Return Time (µs)"=w335:sgl)
            n37 = property class="Camera.lvclass"(reference=w343, "Bit Depth"=w341, "Camera Dimensions"=w340, "Data Representation"=w339, "Duty Cycle"=w338, "Make, Model"=w337, "Max Frequency (kHz)"=w336, "Return Time (µs)"=w335) -> (reference out=w332:refnum<class "Camera.lvclass">)  [unwired: 1 in, 1 out]
            n38 = Bundle By Name(cluster=w334, "Camera out"=w332) -> (w333:T12)
          }
          frame "PC" {
            n39 = local read "PC Ctrl"() -> (w347:T4)
            n40 = Unbundle By Name(w350) -> ("PC out"=w349:refnum<class "PC.lvclass">)
            n41 = Unbundle By Name(w347) -> ("Max Number of Cores"=w346:dbl, "Path to DLL"=w345:path)
            n42 = property class="PC.lvclass"(reference=w349, "Max Number of Cores"=w346, "Path to DLL"=w345) -> (reference out=w348:refnum<class "PC.lvclass">)  [unwired: 1 in, 1 out]
            n43 = Bundle By Name(cluster=w350, "PC out"=w348) -> (w344:T12)
          }
          frame "DAQ" {
            n44 = local read "DAQ Ctrl"() -> (w358:T5)
            n45 = Unbundle By Name(w362) -> ("DAQ out"=w360:refnum<class "DAQ.lvclass">)
            n46 = Unbundle By Name(w358) -> ("Camera Counter"=w357:tag, "Camera Counter PFI"=w356:tag, "Galvo Analog Output Channel(s)"=w355:tag, "Galvo Counter"=w354:tag, "Galvo Counter PFI"=w353:tag, "Master Counter"=w352:tag, "Master Counter PFI"=w351:tag)
            n47 = property class="DAQ.lvclass"(reference=w360, "Camera Counter"=w357, "Camera Counter Output Terminal"=w356, "Galvo Analog Output Channel(s)"=w355, "Galvo Counter"=w354, "Galvo Counter Terminal"=w353, "Master Counter"=w352, "Master Counter Terminal"=w351) -> (reference out=w359:refnum<class "DAQ.lvclass">)  [unwired: 1 in, 1 out]
            n48 = Bundle By Name(cluster=w362, "DAQ out"=w359) -> (w361:T12)
          }
          frame "Laser" {
          }
          frame "Spectrometer" {
            n49 = local read "Spec Ctrl"() -> (w370:T6)
            n50 = Unbundle By Name(w372) -> ("Spectrometer out"=w371:refnum<class "Spectrometer.lvclass">)
            n51 = Unbundle By Name(w370) -> ("Bandwidth (nm)"=w369:dbl, "Center wavelength (nm)"=w368:dbl, "Make Model"=w367:string, "Scan depth (mm)"=w366:dbl)
            n52 = property class="Spectrometer.lvclass"(reference=w371, "Bandwidth (nm)"=w369, "Center wavelength (nm)"=w368, "Make Model"=w367, "Scan depth (mm)"=w366) -> (reference out=w364:refnum<class "Spectrometer.lvclass">)  [unwired: 1 in, 1 out]
            n53 = Bundle By Name(cluster=w372, "Spectrometer out"=w364) -> (w365:T12)
          }
          frame "Galvos" {
            n54 = local read "Galvo Ctrl"() -> (w379:T7)
            n55 = Unbundle(w380) -> (w375:refnum<class "Galvonometer.lvclass">[])  [unwired: 5 out]
            n56 = Unbundle By Name(w379) -> ("Make Model"=w378:string, "Max Scan Angle (degrees)"=w377:dbl, "Output Scale Factor (V/degree)"=w376:dbl)
            n57 = for {
              tunnel: w375 -> [w388] mode=indexing
              tunnel: w378 -> [w387]
              tunnel: w377 -> [w386]
              tunnel: w376 -> [w385]
              tunnel: w375 -> [w383]
              tunnel: [w381] -> w374
              i -> [w384]
              n58 = property class="Galvonometer.lvclass"(reference=w388, "Make Model"=w387, "Max Scan Angle (degrees)"=w386, "Output Scale Factor (V_degrees)"=w385) -> (reference out=w382:refnum<class "Galvonometer.lvclass">)  [unwired: 1 in, 1 out]
              n59 = Replace Array Subset(array=w383, new element=w382, index=w384) -> (w381:refnum<class "Galvonometer.lvclass">[])
            }
            n60 = Bundle(cluster=w380, w374) -> (w373:T12)  [unwired: 5 in]
          }
        }
      }
      frame "Configure Processing" {
        n61 = case shown="\"Dispersion\"" w391 {
          tunnel: w390 -> [w392 w404 w405]
          tunnel: [w392 w393 w405] -> w389
          frame "Display Intensity Mapping", Default {
          }
          frame "Fourier Transform" {
            n62 = local read "Fourier Ctrl"() -> (w401:T9)
            n63 = Unbundle By Name(w404) -> ("Proc out"=w402:refnum<class "ConfigProc.lvclass">)
            n64 = Unbundle By Name(w401) -> ("Blur Coefficient"=w400:dbl, "Blur Int"=w399:dbl, "Cores to Use"=w398:dbl, "Interpolation"=w397:dbl, "Magnification"=w396:dbl, "Power"=w395:dbl, "Soften"=w394:dbl)
            n65 = property class="ConfigProc.lvclass"(reference=w402, "Blur Coefficient"=w400, "Blur Int"=w399, "Cores"=w398, "Interpolation"=w397, "Magnification"=w396, "Power"=w395, "Soften"=w394) -> (reference out=w403:refnum<class "ConfigProc.lvclass">)  [unwired: 1 in, 1 out]
            n66 = Bundle By Name(cluster=w404, "Proc out"=w403) -> (w393:T12)
          }
          frame "Dispersion" {
            # "todo: add these coefficients to the ini\nor change the processing class to include dispersion"
          }
        }
      }
    }
    n67 = Unbundle(w77) -> ("Camera out"=w100:refnum<class "Camera.lvclass">, w99:refnum<class "Galvonometer.lvclass">[])  [unwired: 4 out]
    n68 = local read "Saving"() -> (w85:bool)
    n69 = call "updateScanObj.vi"("Scan Settings"="Scan Settings", "Scan in"=w87) -> ("Scan out"=w89:refnum<class "Scan.lvclass">)  [unwired: 1 in]
    n70 = case shown="True" w85 {
      tunnel: [T15."Enabled" ("Disabled") T15."Enabled" ("Disabled")] -> w78
      frame False {
      }
      frame True {
      }
    }
    n71 = call "ValidateScanInput.vi"("Original Scan"=w87, "New Scan"=w89, "Galvo Array"=w99, "Camera.lvclass"=w100) -> ("Current Scan Schematic"=→"Current Scan Schematic":cluster{dbl[], dbl[]}[], "Max file size exceeded"=w56:bool, "Output scan"=w58:refnum<class "Scan.lvclass">, "Memory (GB)"=→"Memory (GB)":dbl, "Time (s)"=→"Time (s)":sgl, "Max Voltage Exceeded"=→"Exceeds Max Voltage":bool)
    "Max file size exceeded" <- w56
    n72 = case shown="False" w56 {
      tunnel: [T15."Enabled" ("Disabled") T15."Disabled and Grayed Out" ("Disabled")] -> w55
      frame False {
      }
      frame True {
      }
    }
    n73 = control-ref of="Pane"() -> (w73:refnum<vi>)
    n74 = property class="Scan.lvclass"(reference=w58) -> ("X FOV (degrees)"=w84:dbl, "Y FOV (degrees)"=w83:dbl)  [unwired: 1 in, 2 out]
    n75 = control-ref of="Save"() -> (w54:refnum<vi>)
    n76 = property on="X FOV (°)" class="DigNum (strict)"("Value"=w84) -> ()  [unwired: 2 in, 2 out]
    n77 = property class="Bool (strict)"(reference=w54, "DisabledEnum"=w55) -> (error out=w53:errorcluster)  [unwired: 1 in, 1 out]
    n78 = property class="Pane"(reference=w73, error in=w53) -> ("Controls[]"=w72:refnum<vi>[])  [unwired: 2 out]
    n79 = for {
      tunnel: w72 -> [w327] mode=indexing
      tunnel: w78 -> [w326]
      n80 = property class="Ctl"(reference=w327, "DisabledEnum"=w326) -> ()  [unwired: 1 in, 2 out]
    }
    n81 = property on="Y FOV (°)" class="DigNum (strict)"("Value"=w83) -> ()  [unwired: 2 in, 2 out]
    n82 = case shown="True" "Save Settings" {
      selector: "Save Settings" -> [_ w323]
      tunnel: w77 -> [w321 w325]
      tunnel: [w321 w324] -> w76
      tunnel: [FALSE w322] -> w74
      frame False {
      }
      frame True {
        n83 = Not(x=w323) -> (.not. x?=w322:bool)
        n84 = call "write_ini.vi"("Current OCT settings"=w325) -> ("OCT settings out"=w324:T16)
      }
    }
    n85 = local write "Save Settings"(w74) -> ()
    n86 = local write "Stopping"(w74) -> ()
    n87 = flat-sequence {
      tunnel: w76 -> [w119]
      tunnel: w58 -> [w105]
      tunnel: [w122] -> w96
      tunnel: [w120] -> w95
      tunnel: [w118] -> w94
      tunnel: [w105] -> w93
      tunnel: [w115] -> w92
      tunnel: [w117] -> w91
      tunnel: [w130] -> w71
      tunnel: [w143] -> w69
      tunnel: [w137] -> w67
      tunnel: [w142] -> w64
      tunnel: w91 -> [w137]
      tunnel: w92 -> [w131]
      tunnel: w93 -> [w142]
      tunnel: w94 -> [w128]
      tunnel: w95 -> [w129]
      tunnel: w96 -> [w140]
      tunnel: [w136] -> w62
      tunnel: [w128] -> w61
      tunnel: [w135] -> w60
      tunnel: [w134] -> w59
      tunnel: w71 -> [w267]
      tunnel: [w271] -> w70
      tunnel: w69 -> [w265]
      tunnel: [w259] -> w68
      tunnel: w67 -> [w273]
      tunnel: [w273] -> w66
      tunnel: [w272] -> w65
      tunnel: w64 -> [w270]
      tunnel: [w270] -> w63
      tunnel: w62 -> [w272]
      tunnel: w61 -> [w266]
      tunnel: w60 -> [w269]
      tunnel: w59 -> [w268]
      tunnel: [w258] -> w51
      tunnel: w70 -> [w311]
      tunnel: w68 -> [w310]
      tunnel: w66 -> [w315]
      tunnel: w65 -> [w314]
      tunnel: w63 -> [w313]
      tunnel: [w313] -> w88
      tunnel: [w301] -> w52
      tunnel: w51 -> [w300]
      tunnel: [w300] -> w50
      frame #0 {
        # "Initialization and preallocation"
        n88 = Unbundle(w119) -> ("Def Camera"=w110:refnum<class "Camera.lvclass">, "Def DAQ"=w124:refnum<class "DAQ.lvclass">, "Array"=w109:refnum<class "Galvonometer.lvclass">[])  [unwired: 3 out]
        n89 = local read "Saving"() -> (w116:bool)
        n90 = call "GetRaster.vi"("Scan in"=w105, "Camera in"=w110, "Galvo Array"=w109, "error in (no error)"=errorcluster {"status"=FALSE, "code"=0, "source"=""}) -> ("Return A"=w106:dbl, "cropLinesOut"=w103:dbl, "Delay A"=w104:dbl, "Galvo Array"=w108:dbl[][], "error IO"=w107:errorcluster)
        "cropLinesOut" <- w103
        n91 = control-ref of="Progress"() -> (w111:refnum<vi>)
        n92 = call "SyncGalvosCamera.vi"("Camera in"=w110, "DAQ in"=w124, "Return A"=w106, "error in (no error)"=w107, "Scan in"=w105, "Galvo Array"=w109, "Raster"=w108, "Crop A"=w103, "Settling A"=w104) -> ("Sync Err Out"=w121:errorcluster, "DAQ out"=w114:refnum<class "DAQ.lvclass">)
        n93 = call "createQueues.vi"() -> ("Display Queue"=w117:refnum<queue>)  [unwired: 5 in]
        n94 = call "PreallocateArraysFFTW3.vi"("Camera.lvclass"=w110, "Scan.lvclass"=w105) -> ("FFTW3 input"=w122:T17)
        n95 = call "InitCameraSeq.vi"("Saving"=w116, "Scan.lvclass"=w105, "error in"=w121, "Progress"=w111, "cropLines"=w103, "DAQ in"=w114) -> ("error out"=w120:errorcluster, "Stop out"=w112:bool, "Updated camera"=w115:T19, "DAQ out"=w113:refnum<class "DAQ.lvclass">)  [unwired: 1 in]
        n96 = Bundle By Name(cluster=w119, "Def DAQ"=w113) -> (w118:T16)
        n97 = local write "Reset"(w112) -> ()
      }
      frame #1 {
        # "Aim loops"
        n98 = Unbundle By Name(w128) -> ("Def Proc"=w139:refnum<class "ConfigProc.lvclass">, "Def Spectrometer"=w138:refnum<class "Spectrometer.lvclass">)
        n99 = Unbundle(w140) -> (w141:dbl[][])  [unwired: 3 out]
        n100 = Unbundle By Name(w131) -> ("IMAQ Session Out"=w132:refnum<k11>, "New Image"=w133:T18)
        n101 = local read "wavenumber vector"() -> (w126:dbl[])
        n102 = local read "P"() -> (w125:dbl[])
        n103 = local read "Gc"() -> (w127:cdb[])
        n104 = while {
          tunnel: w140 -> [w166]
          shift-right: [w164] -> w135
          shift-left: w141 -> [w165]
          tunnel: w139 -> [w161]
          tunnel: w138 -> [w160]
          tunnel: w137 -> [w155]
          tunnel: w142 -> [w159]
          tunnel: [w151] -> w134
          shift-right: [w146] -> w136
          shift-left: w129 -> [w150]
          shift-right: [w148] -> _
          shift-left: w127 -> [w147]
          tunnel: w126 -> [w145]
          tunnel: w125 -> [w144]
          stop <- w156 stop-if-true
          # "Process/Display loop"
          n105 = local read "cropLinesOut"() -> (w149:dbl)
          n106 = local read "Saving"() -> (w154:bool)
          n107 = Dequeue Element(queue=w155, timeout in ms (-1)=100) -> (element=w163:u16[][], timed out?=w153:bool)  [unwired: 1 in, 2 out]
          n108 = Or(x=w154, y=w153) -> (x .or. y?=w152:bool)
          n109 = case shown="False" w152 {
            tunnel: w166 -> [w189 w241]
            tunnel: w165 -> [w188 w242]
            tunnel: [w187 w242] -> w164
            tunnel: w163 -> [w181 _]
            tunnel: w161 -> [w186 _]
            tunnel: w160 -> [w185 _]
            tunnel: w159 -> [w180 _]
            tunnel: [w183 w241] -> w151
            tunnel: w150 -> [w174 w239]
            tunnel: w149 -> [w179 _]
            tunnel: [w170 w240] -> w148
            tunnel: w147 -> [w172 w240]
            tunnel: [w169 w239] -> w146
            tunnel: w145 -> [w168 _]
            tunnel: w144 -> [w167 _]
            frame False {
              # "No buffer timeout"
              n110 = local read "Optimize DispComp"() -> (w175:bool)
              n111 = call "cropInactive.vi"("Scan in"=w180, "Whole camera frame"=w181, "cropLines"=w179) -> ("Cropped camera frame"=w176:u16[][])  [unwired: 1 in]
              n112 = call "line_spectrum.vi"("Image"=w176) -> ("Mean intensity per pixel"=→"Mean intensity per pixel":cluster{"Ramp Pattern":dbl[], dbl[]}[])
              n113 = case shown="True" w175 {
                selector: w175 -> [_ w202]
                tunnel: w176 -> [_ w203]
                tunnel: w174 -> [w191 w200]
                tunnel: [w191 w199] -> w173
                tunnel: [w190 w194] -> w171
                tunnel: w172 -> [w190 _]
                tunnel: w168 -> [_ w193]
                tunnel: w167 -> [_ w192]
                frame False {
                }
                frame True {
                  # "on optimize press"
                  n114 = local read "Dispersion Ctrl"() -> (w198:cluster{"C2":dbl, "C3":dbl})
                  n115 = Not(x=w202) -> (.not. x?=w201:bool)
                  n116 = call "call_opt_DispComp_matlab.vi"("error in"=w200, "Wavenumber"=w193, "P"=w192, "Raw image"=w203) -> ("error out"=w199:errorcluster, "C3 out"=w196:dbl, "C2 out"=w197:dbl, "dispCompPhasor"=w194:cdb[])  [unwired: 4 in]
                  n117 = local write "Optimize DispComp"(w201) -> ()
                  n118 = Bundle By Name(cluster=w198, "C2"=w197, "C3"=w196) -> (w195:cluster{"C2":dbl, "C3":dbl})
                  n119 = local write "Dispersion Ctrl"(w195) -> ()
                  n120 = local write "Gc"(w194) -> ()
                }
              }
              n121 = local read "Skip FFT"() -> (w184:bool)
              n122 = case shown="False" w184 {
                tunnel: w189 -> [w216 w236]
                tunnel: w188 -> [w215 w237]
                tunnel: [w214 w237] -> w187
                tunnel: [w213 w238] -> w182
                tunnel: w176 -> [w210 w238]
                tunnel: w186 -> [w212 _]
                tunnel: w185 -> [_ _]
                tunnel: [w208 w236] -> w183
                tunnel: w173 -> [w211 w234]
                tunnel: w171 -> [w209 w235]
                tunnel: [w206 w235] -> w170
                tunnel: [w207 w234] -> w169
                tunnel: w168 -> [w205 _]
                tunnel: w167 -> [w204 _]
                frame False {
                  # "do OCT"
                  n123 = disable-structure shown="Enabled" {
                    disable-tunnel: w216 -> [w225 w229]
                    disable-tunnel: w215 -> [w224 w230]
                    disable-tunnel: [w223 w230] -> w214
                    disable-tunnel: [w222 w231] -> w213
                    disable-tunnel: w212 -> [w221 _]
                    disable-tunnel: w211 -> [w220 w228]
                    disable-tunnel: w210 -> [w219 w232]
                    disable-tunnel: w205 -> [w218 w233]
                    disable-tunnel: w209 -> [w217 w227]
                    disable-tunnel: [_ w229] -> w208
                    disable-tunnel: [_ w228] -> w207
                    disable-tunnel: [w217 w227] -> w206
                    disable-tunnel: w204 -> [_ w226]
                    frame Disabled {
                      n124 = call "getIFT_callDLL.vi"("Processing Configuration"=w221, "FFTW3 arrays"=w225, "Buffer in"=w224, "error in (no error)"=w220, "Interferogram"=w219, "Spectrum calibration"=w218) -> ("Depth Profile"=w222:dbl[][], "Buffer out"=w223:dbl[][])  [unwired: 10 in, 2 out]
                    }
                    frame Enabled {
                      # "LV parallel processing with dispComp"
                      n125 = call "processFrame.vi"("Image"=w232, "Gc"=w227, "wavenumber vector"=w233, "P"=w226) -> ("Image out"=w231:dbl[][])  [unwired: 7 in]
                    }
                  }
                }
                frame True {
                  # "show raw camera image"
                }
              }
              n126 = call "flipAndAverageBidirectional.vi"("Depth"=w182) -> ("Depth out"=→"Depth":dbl[][])  [unwired: 2 in]
            }
            frame True {
              # "Skip on buffer timeout or saving"
            }
          }
          n127 = local read "Saving"() -> (w158:bool)
          n128 = local read "Stopping"() -> (w157:bool)
          n129 = Or(x=w158, y=w157) -> (x .or. y?=w156:bool)
        }
        n130 = while {
          tunnel: [w257] -> w143
          tunnel: w129 -> [w256]
          tunnel: w137 -> [w255]
          tunnel: w133 -> [w245]
          tunnel: w132 -> [w244]
          tunnel: w131 -> [w243]
          tunnel: [w243] -> w130
          stop <- w248 stop-if-true
          # "Acquire loop"
          n131 = local read "Saving"() -> (w247:bool)
          n132 = local read "Save Settings"() -> (w250:bool)
          n133 = local read "Reset"() -> (w254:bool)
          n134 = local read "Save"() -> (w253:bool)
          n135 = local read "Stop"() -> (w252:bool)
          n136 = Compound Arithmetic op=OR(w253, w254, w252, w250) -> (w246:bool)
          n137 = call "GrabFrame.vi"("IMAQ Session Out"=w244, "error in"=w256, "Stop"=w246, "Saving"=w247, "New Image"=w245) -> ("error out"=w257:errorcluster, "Stopped"=w249:bool, "Image Pixels (U16)"=w251:u16[][])  [unwired: 1 in]
          n138 = Or(x=w249, y=w247) -> (x .or. y?=w248:bool)
          "Stopping" <- w248
          n139 = Enqueue Element(queue=w255, element=w251) -> ()  [unwired: 2 in, 3 out]
        }
      }
      frame #2 {
        # "Stop Scanners & Camera, Write files"
        n140 = local read "Saving"() -> (w262:bool)
        n141 = call "closeImaqSession.vi"("error in"=w265, "Updated camera"=w267, "Saving"=w262) -> ("error out"=w261:errorcluster, "Updated camera out"=w264:T20)  [unwired: 7 in]
        n142 = case shown="True" w262 {
          tunnel: w264 -> [w276 w284]
          tunnel: [w276 w281] -> w271
          tunnel: [w275 w285] -> w260
          tunnel: w266 -> [w274 w283]
          tunnel: w270 -> [_ w282]
          tunnel: w269 -> [_ w288]
          tunnel: w268 -> [_ w289]
          tunnel: w261 -> [w275 w292]
          tunnel: [w274 w283] -> w258
          frame False {
          }
          frame True {
            n143 = local read "File Ctrl"() -> (w291:T10)
            n144 = local read "cropLinesOut"() -> (w278:dbl)
            n145 = local read "Memory (GB)"() -> (w277:dbl)
            n146 = local read "Skip Processing"() -> (w279:bool)
            n147 = control-ref of="Progress"() -> (w280:refnum<vi>)
            n148 = call "writeToBinary.vi"("cropLinesOut"=w278, "File control"=w291, "Scan"=w282, "Memory (GB)"=w277, "Updated camera"=w284, "error in"=w292, "Progress"=w280) -> ("Output Path"=w287:path, "OCT filename out"=w286:string, "Camera out"=w281:T20, "error out"=w290:errorcluster)  [unwired: 5 in]
            n149 = case shown="False" w279 {
              tunnel: w290 -> [_ w299]
              tunnel: w289 -> [_ _]
              tunnel: w288 -> [_ _]
              tunnel: w287 -> [w298 _]
              tunnel: w286 -> [w297 _]
              tunnel: [_ w299] -> w285
              tunnel: w282 -> [_ _]
              tunnel: w281 -> [w296 _]
              tunnel: w280 -> [_ _]
              tunnel: w278 -> [_ _]
              frame False {
                n150 = local read "Dispersion Ctrl"() -> (w295:cluster{"C2":dbl, "C3":dbl})
                n151 = Unbundle(w295) -> ("C2"=w294:dbl, "C3"=w293:dbl)
                n152 = call "processOctaVolMatlab.vi"("C2"=w294, "Output Path"=w298, "C3"=w293, "Updated camera"=w296, "OCT filename out"=w297) -> ()  [unwired: 11 in]
              }
              frame True {
              }
            }
          }
        }
        n153 = Unbundle By Name(w258) -> ("Def DAQ"=w263:refnum<class "DAQ.lvclass">)
        n154 = call "stopAllTasks.vi"("error in"=w260, "DAQ in"=w263) -> ("error out"=w259:errorcluster)  [unwired: 1 out]
      }
      frame #3 {
        w312 = FALSE
        # "Reset stop buttons"
        # "Close files, flush queues, clear memory, reset"
        n155 = local read "Saving"() -> (w305:bool)
        n156 = call "CloseCamera.vi"("error in"=w310, "Updated camera"=w311, "Saving"=w305) -> ("error out"=w308:errorcluster, "Saving out"=w304:bool)  [unwired: 1 in]
        n157 = local read "Save"() -> (w309:bool)
        n158 = local write "Saving"(w304) -> ()
        n159 = Flush Queue(queue=w315, error in (no error)=w308) -> (error out=w307:errorcluster)  [unwired: 2 out]
        n160 = local write "Stopping"(w312) -> ()
        n161 = local write "Reset"(w312) -> ()
        n162 = Merge Errors(w307, w314) -> (w306:errorcluster)
        n163 = call <vilib>:"Simple Error Handler.vi"("error in (no error)"=w306) -> ("error out"=w303:errorcluster)  [unwired: 4 in, 4 out]
        n164 = case shown="False" w309 {
          tunnel: w303 -> [w316 w317]
          tunnel: [w316 w317] -> w302
          frame False {
            # "Do nothing"
          }
          frame True {
            # "Set Saving to true for next iteration"
            n165 = local write "Save"(FALSE ("Save")) -> ()
            n166 = local write "Saving"(TRUE) -> ()
          }
        }
        "Other error" <- w302
        n167 = local read "Stop"() -> (w301:bool)
      }
    }
  }
  n168 = Not(x=w1) -> (.not. x?=w2:bool)
  n169 = local write "Stop"(w2) -> ()
